vi "MoveJudge.vi"(8 "LowComm":string, 9 "UpComm":string, 11 "Command In":string) -> (2 "Move":string, 3 "Command Out":string)   [LabVIEW 2016]
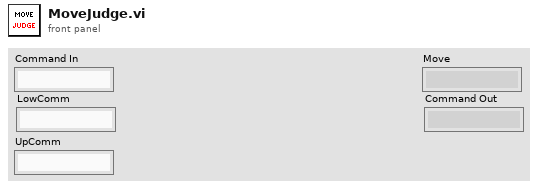
[diagram p1: front panel]
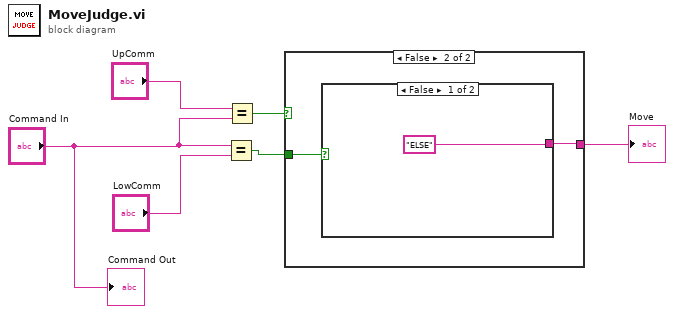
[diagram p0: block diagram]
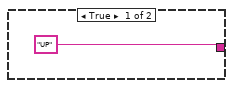
[diagram p2: hidden frame]
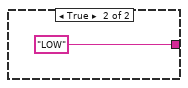
[diagram p3: hidden frame]
diagram:
  n1 = Equal?(x="Command In", y="LowComm") -> (x = y?=w3:bool)
  n2 = Equal?(x="UpComm", y="Command In") -> (x = y?=w4:bool)
  n3 = case shown="False" w4 {
    tunnel: w3 -> [_ w9]
    tunnel: ["UP" w8] -> w2
    frame True {
    }
    frame False {
      n4 = case shown="False" w9 {
        tunnel: ["ELSE" "LOW"] -> w8
        frame False {
        }
        frame True {
        }
      }
    }
  }
  "Move" <- w2
  "Command Out" <- "Command In"
